vi "Init.vi"(8 "error in (no error)":errorcluster, 11 "VI Refnum":refnum<vi>) -> (0 "error out":errorcluster)   [LabVIEW 2013, in "main.lvlib"]
uses:
  main.lvlib
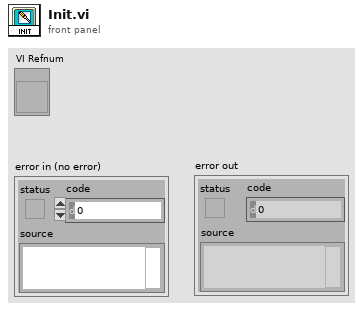
[diagram p1: front panel]
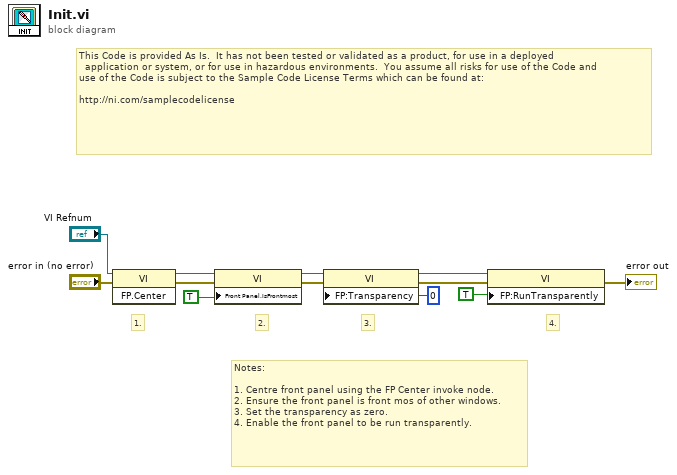
[diagram p0: block diagram]
diagram:
  # "This Code is provided As Is.  It has not been tested or validated as a product, for use in a deployed\n  application or system, or for use in hazardous environments.  You assume all risks for use of the Code and   \nuse of the Code is subject to the Sample Code License Terms which can be found at: \n\nhttp://ni.com/samplecodelicense"
  # "Notes:\n\n1. Centre front panel using the FP Center invoke node.\n2. Ensure the front panel is front mos of other windows.\n3. Set the transparency as zero.\n4. Enable the front panel to be run transparently."
  # "4."
  # "3."
  # "2."
  # "1."
  n1 = invoke class="VI" method="FP.Center"(reference="VI Refnum", error in="error in (no error)") -> (reference out=w5:refnum<vi>, error out=w4:errorcluster)  [unwired: 1 in, 1 out]
  n2 = property class="VI"("Front Panel.IsFrontmost"=TRUE ("Front Panel Window:Run VI Transparently")) -> ()  [unwired: 2 in, 2 out]
  n3 = property class="VI"(reference=w5, error in=w4, "FP:Transparency"=u8 0 ("Front Panel Window:Transparency")) -> (reference out=w2:refnum<vi>, error out=w3:errorcluster)
  n4 = property class="VI"(reference=w2, error in=w3, "FP:RunTransparently"=TRUE ("Front Panel Window:Run VI Transparently")) -> (error out=→"error out":errorcluster)  [unwired: 1 out]
